vi "Close.vi"(8 "error in (no error)":errorcluster, 11 "Simulate in":refnum<class "Simulated DMM.lvclass">) -> (0 "error out":errorcluster, 2 "Result Text":string="PCI-4070 has been initialized", 3 "Simulate out":refnum<class "Simulated DMM.lvclass">)   [LabVIEW 2012, in "Simulated DMM.lvclass"]
uses:
  Simulated DMM.lvclass
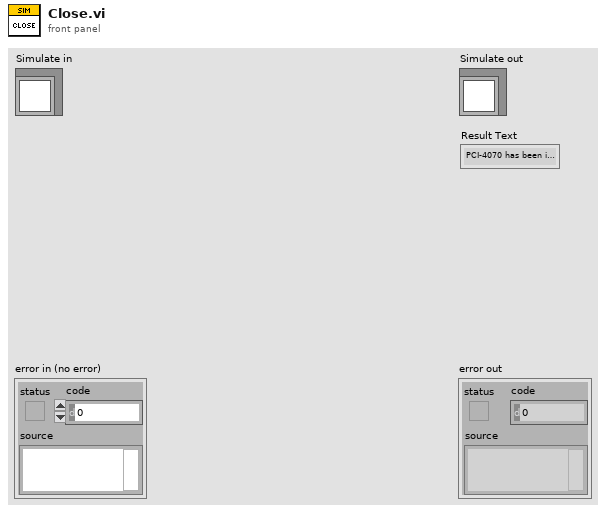
[diagram p1: front panel]
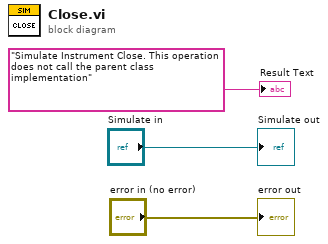
[diagram p0: block diagram]
diagram:
  "error out" <- "error in (no error)"
  "Simulate out" <- "Simulate in"
  "Result Text" <- "Simulate Instrument Close. This operation does not call the parent class implementation" ("message")
